vi "test Copy Blob.vi"(8 "error in (no error)":errorcluster, 11 "TestCase in":refnum<class "Test_Blob.lvclass">) -> (0 "error out":errorcluster, 3 "TestCase out":refnum<class "Test_Blob.lvclass">)   [LabVIEW 2015, in "Test_Blob.lvclass"]
uses:
  Test_Blob.lvclass
  Blob Storage/Blob Type.ctl
  Global Parameters.vi
  Core/Session/Session.lvclass
  Blob Storage/NI_Azure_Blob.lvlib
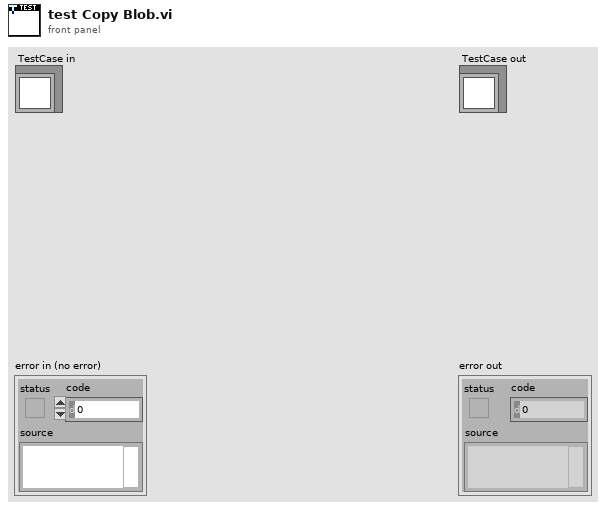
[diagram p1: front panel]
types:
  T1 = typedef "NI_Azure_Blob.lvlib/Blob Type.ctl" = enum16{"BlockBlob", "PageBlob", "AppendBlob"}
  T2 = typedef "NI_Azure_Core.lvlib/Session.lvclass/Azure Credentials.ctl" = cluster{"Storage Account Name":string, "Access Key":string}
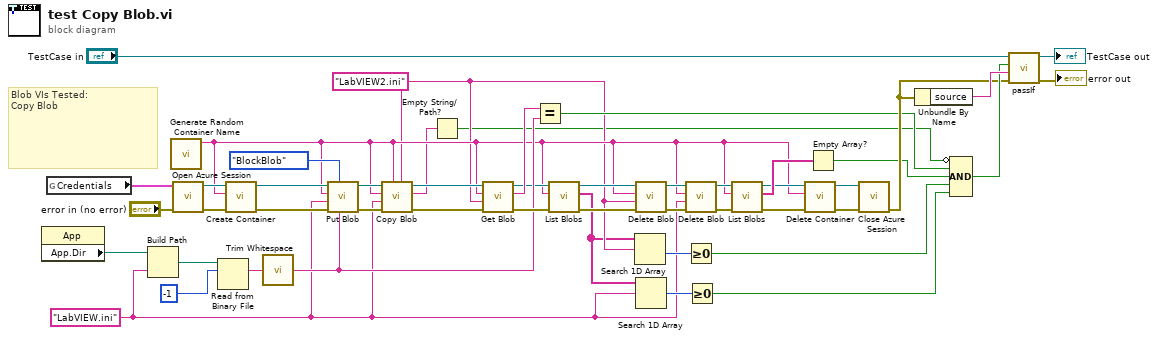
[diagram p0: block diagram]
diagram:
  w8 = "LabVIEW2.ini"
  w3 = "LabVIEW.ini"
  # "Blob VIs Tested:\nCopy Blob"
  n1 = property class="App"() -> ("App.Dir"=w44:path)  [unwired: 2 in, 2 out]
  n2 = global read "Global Parameters.vi" "Credentials"() -> (w28:T2)
  n3 = Build Path(base path=w44, name or relative path=w3) -> (appended path=w43:path)
  n4 = call "Generate Random Container Name.vi"() -> ("Random Container Name"=w9:string)  [unwired: 11 in]
  n5 = call "Open Azure Session.vi"("error in (no error)"="error in (no error)", "Credentials"=w28) -> ("error out"=w29:errorcluster, "Azure Session"=w25:refnum<class "Session.lvclass">)  [unwired: 8 in]
  n6 = Read from Binary File(10:-1 ("count (1)"), 11:w43) -> (2:w37:string)  [unwired: 4 in, 3 out]
  n7 = call "Create Container.vi"("error in (no error)"=w29, "Container"=w9, "Azure Session in"=w25) -> ("error out"=w41:errorcluster, "Azure Session out"=w40:refnum<class "Session.lvclass">)  [unwired: 7 in]
  n8 = call <vilib>:"Trim Whitespace.vi"("string"=w37) -> ("trimmed string"=w18:string)  [unwired: 1 in]
  n9 = call "Put Blob.vi"("Blob Content"=w18, "Blob type"=Blob_Type."BlockBlob", "error in (no error)"=w41, "Blob"=w3, "Container"=w9, "Azure Session in"=w40) -> ("error out"=w39:errorcluster, "Azure Session out"=w38:refnum<class "Session.lvclass">)  [unwired: 4 in]
  n10 = call "Copy Blob.vi"("Destination Blob"=w8, "Destination Container"=w9, "error in (no error)"=w39, "Source Blob"=w3, "Source Container"=w9, "Azure Session in"=w38) -> ("error out"=w36:errorcluster, "Copy ID"=w2:string, "Azure Session out"=w20:refnum<class "Session.lvclass">)  [unwired: 3 in]
  n11 = Empty String/Path?(string/path=w2) -> (empty?=w1:bool)
  n12 = call "Get Blob.vi"("error in (no error)"=w36, "Blob"=w8, "Container"=w9, "Azure Session in"=w20) -> ("error out"=w21:errorcluster, "Blob Content"=w19:string, "Azure Session out"=w14:refnum<class "Session.lvclass">)  [unwired: 5 in]
  n13 = Equal?(x=w19, y=w18) -> (x = y?=w16:bool)
  n14 = call "List Blobs.vi"("error in (no error)"=w21, "Container"=w9, "Azure Session in"=w14) -> ("error out"=w15:errorcluster, "Blobs"=w6:string[], "Azure Session out"=w11:refnum<class "Session.lvclass">)  [unwired: 6 in]
  n15 = Search 1D Array(1D array=w6, element=w8) -> (index of element=w7:i32)  [unwired: 1 in]
  n16 = call "Delete Blob.vi"("error in (no error)"=w15, "Blob"=w8, "Container"=w9, "Azure Session in"=w11) -> ("error out"=w12:errorcluster, "Azure Session out"=w10:refnum<class "Session.lvclass">)  [unwired: 6 in]
  n17 = Search 1D Array(1D array=w6, element=w3) -> (index of element=w5:i32)  [unwired: 1 in]
  n18 = call "Delete Blob.vi"("error in (no error)"=w12, "Blob"=w3, "Container"=w9, "Azure Session in"=w10) -> ("error out"=w35:errorcluster, "Azure Session out"=w34:refnum<class "Session.lvclass">)  [unwired: 6 in]
  n19 = Greater Or Equal To 0?(x=w7) -> (x >= 0?=w13:bool)
  n20 = Greater Or Equal To 0?(x=w5) -> (x >= 0?=w4:bool)
  n21 = call "List Blobs.vi"("error in (no error)"=w35, "Container"=w9, "Azure Session in"=w34) -> ("error out"=w32:errorcluster, "Blobs"=w33:string[], "Azure Session out"=w31:refnum<class "Session.lvclass">)  [unwired: 6 in]
  n22 = call "Delete Container.vi"("error in (no error)"=w32, "Container"=w9, "Azure Session in"=w31) -> ("error out"=w27:errorcluster, "Azure Session out"=w22:refnum<class "Session.lvclass">)  [unwired: 7 in]
  n23 = Empty Array?(array=w33) -> (empty?=w17:bool)
  n24 = call "Close Azure Session.vi"("error in (no error)"=w27, "Azure Session"=w22) -> ("error out"=w23:errorcluster)  [unwired: 9 in]
  n25 = Unbundle By Name(w23) -> ("source"=w45:string)
  n26 = Compound Arithmetic op=AND(invert w1, w16, w17, w13, w4) -> (w26:bool)
  n27 = call-dynamic "passIf.vi"("error in (no error)"=w23, "message (\"\")"=w45, "pass"=w26, "TestCase in"="TestCase in") -> ("error out"=→"error out":errorcluster, "TestCase out"=→"TestCase out":refnum<class "Test_Blob.lvclass">)  [unwired: 6 in]
